vi "DetectCamera.vi"(8 "error in (no error)":errorcluster, 11 "Config In":T1) -> (0 "error out":errorcluster, 3 "Config Out":T1)   [LabVIEW 2019]
uses:
  Settings/Settings.ctl
  Support/Hardware Configuration.ctl
  Acquisition/Signal Type.ctl
  Logging/Logging Configuration.ctl
  Support/Camera Configuration.ctl
  E:/DevHardSoftware/MMicroscopy/HardwareAdapter/Camera/Dependencies/PVCamNET.dll
  Dependencies/PVCamNET.dll
  Acquisition/Acquisition.lvlib
  Logging/Logging.lvlib
  Settings/Settings.lvlib
panel:
  in  "Exposure time":dbl=30.0
  in  "stop":bool
  in  "start":bool
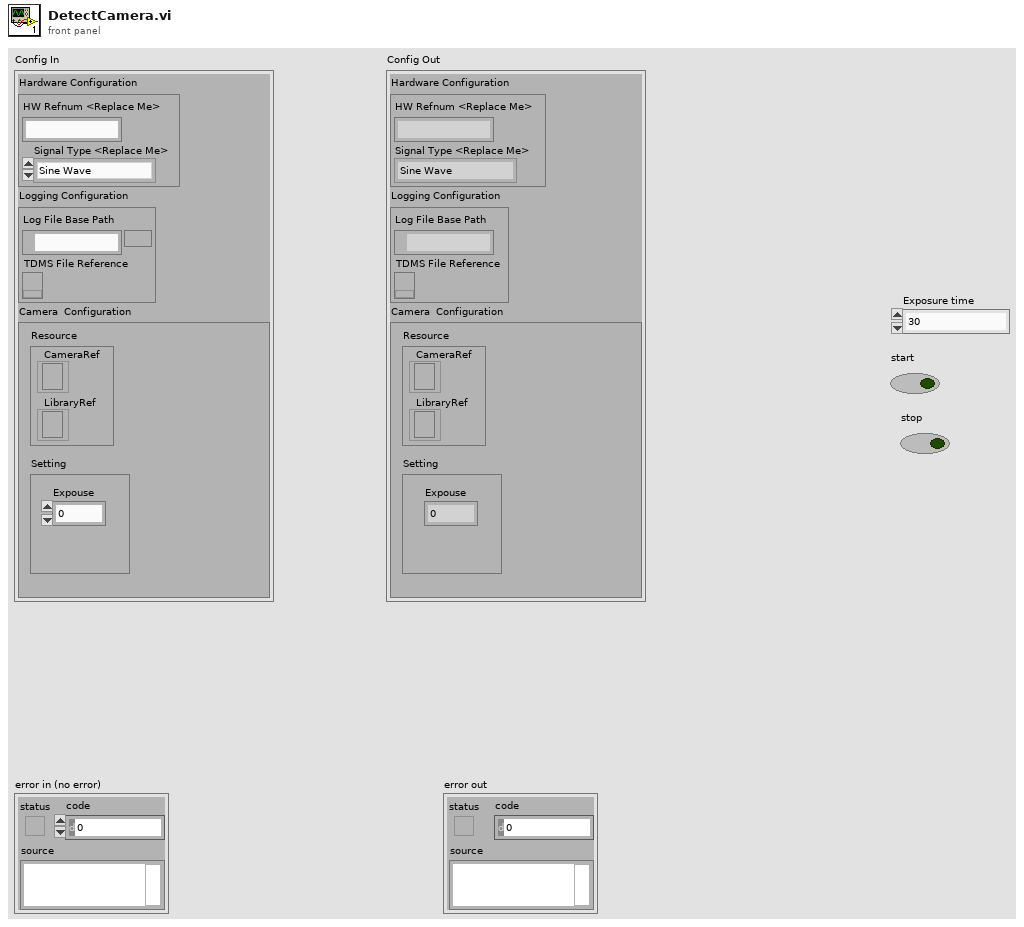
[diagram p1: front panel]
types:
  T1 = typedef "Settings.lvlib/Settings.ctl" = cluster{"Hardware Configuration":T2, "Logging Configuration":T4, "Camera Configuration":T5}
  T2 = typedef "Hardware Configuration.ctl" = cluster{"HW Refnum <Replace Me>":string, "Signal Type <Replace Me>":T3}
  T3 = typedef "Acquisition.lvlib/Signal Type.ctl" = enum16{"Sine Wave", "Square with Noise"}
  T4 = typedef "Logging.lvlib/Logging Configuration.ctl" = cluster{"Log File Base Path":path, "TDMS File Reference":refnum<k34>}
  T5 = typedef "Camera Configuration.ctl" = cluster{"Resource":cluster{"CameraRef":refnum<k24>, "LibraryRef":refnum<k24>}, "Setting":cluster{"Expouse":dbl}}
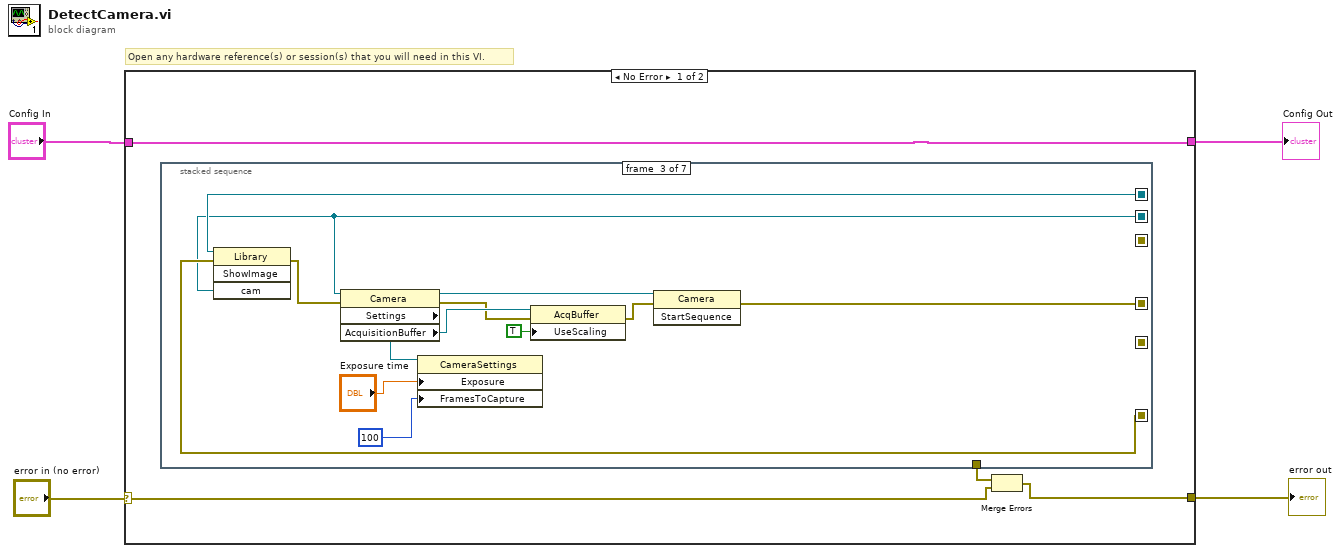
[diagram p0: block diagram]
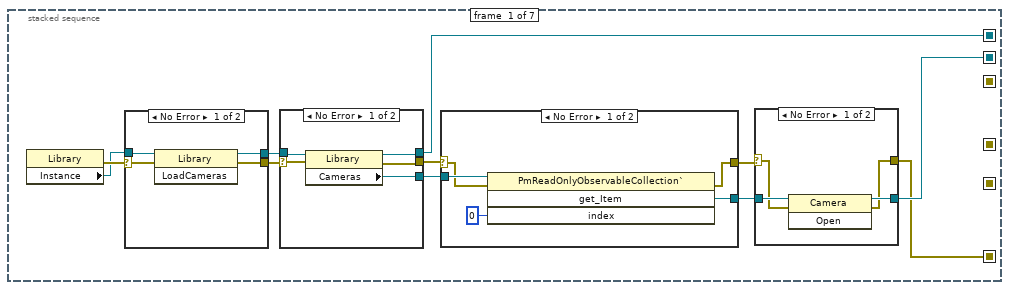
[diagram p2: hidden frame]
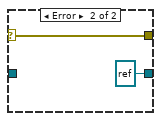
[diagram p3: hidden frame]
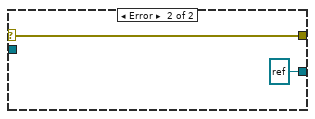
[diagram p4: hidden frame]
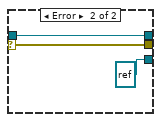
[diagram p5: hidden frame]
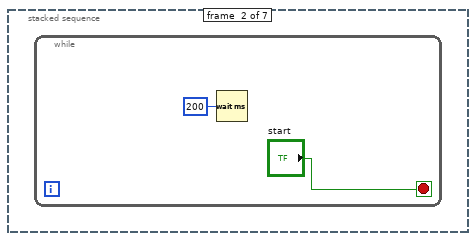
[diagram p7: hidden frame]
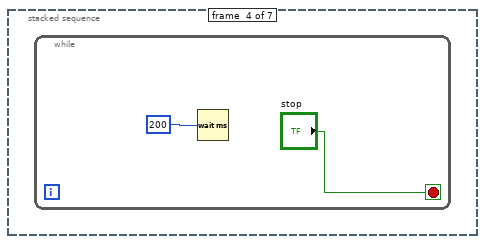
[diagram p8: hidden frame]
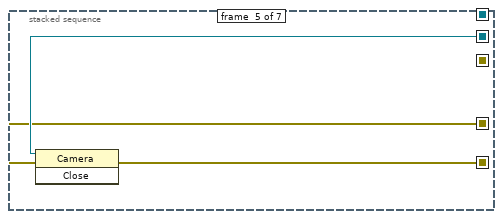
[diagram p9: hidden frame]
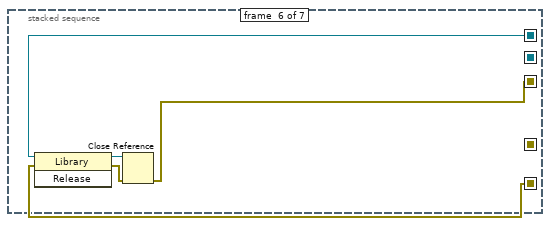
[diagram p10: hidden frame]
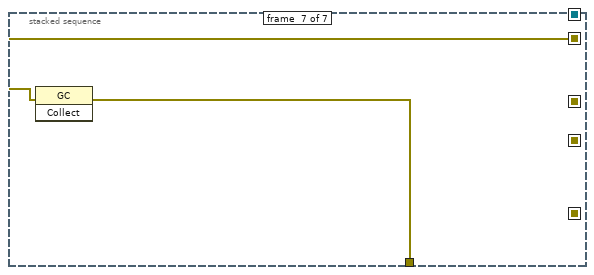
[diagram p11: hidden frame]
diagram:
  # "Open any hardware reference(s) or session(s) that you will need in this VI."
  n1 = case shown="No Error" "error in (no error)" {
    selector: "error in (no error)" -> [w6 w74]
    tunnel: [w5 w74] -> w3
    tunnel: "Config In" -> [w8 w75]
    tunnel: [w8 w75] -> w1
    frame No Error {
      n2 = stacked-sequence {
        seq-local: [w9 _ _ _ _ _ _] -> [_ _ w55 _ _ _ _]
        seq-local: [w10 _ _ _ _ _ _] -> [_ _ w53 _ w66 _ _]
        seq-local: [w11 _ _ _ _ _ _] -> [_ _ w61 _ _ w70 _]
        seq-local: [_ _ w49 _ _ _ _] -> [_ _ _ _ w65 _ _]
        seq-local: [_ _ _ _ w64 _ _] -> [_ _ _ _ _ w69 _]
        seq-local: [_ _ _ _ _ w67 _] -> [_ _ _ _ _ _ w73]
        tunnel: [_ _ _ _ _ _ w72] -> w7
        frame #0 {
          n3 = property class="Library"() -> (error out=w19:errorcluster, "Instance"=w16:refnum<k24>)  [unwired: 2 in, 1 out]
          n4 = case shown="No Error" w19 {
            selector: w19 -> [w42 w46]
            tunnel: [w43 w46] -> w17
            tunnel: [w44 w45] -> w18
            tunnel: w16 -> [w41 w45]
            frame No Error {
              n5 = invoke class="Library" method="LoadCameras"(reference=w41, error in=w42) -> (reference out=w44:refnum<k24>, error out=w43:errorcluster)  [unwired: 1 in, 1 out]
            }
            frame Error {
            }
          }
          n6 = case shown="No Error" w17 {
            selector: w17 -> [w37 w40]
            tunnel: [w34 w40] -> w13
            tunnel: w18 -> [w36 w39]
            tunnel: [w35 w39] -> w11
            tunnel: [w33 refnum<k24> refnum ("Cameras")] -> w15
            frame No Error {
              n7 = property class="Library"(reference=w36, error in=w37) -> (reference out=w35:refnum<k24>, error out=w34:errorcluster, "Cameras"=w33:refnum<k24>)
            }
            frame Error {
            }
          }
          n8 = case shown="No Error" w13 {
            selector: w13 -> [w27 w32]
            tunnel: w15 -> [w30 _]
            tunnel: [w28 refnum<k24> refnum ("get_Item")] -> w14
            tunnel: [w26 w32] -> w12
            frame No Error {
              n9 = invoke class="PmReadOnlyObservableCollection`" method="get_Item"(reference=w30, error in=w27, "index"=0) -> (error out=w26:errorcluster, "get_Item"=w28:refnum<k24>)  [unwired: 1 in, 2 out]
            }
            frame Error {
            }
          }
          n10 = case shown="No Error" w12 {
            selector: w12 -> [w21 w25]
            tunnel: [w20 w25] -> w9
            tunnel: w14 -> [w23 _]
            tunnel: [w22 refnum<k24> refnum ("get_Item")] -> w10
            frame No Error {
              n11 = invoke class="Camera" method="Open"(reference=w23, error in=w21) -> (reference out=w22:refnum<k24>, error out=w20:errorcluster)  [unwired: 1 in, 1 out]
            }
            frame Error {
            }
          }
        }
        frame #1 {
          n12 = while {
            stop <- "start" stop-if-true
            n13 = Wait (ms)(milliseconds to wait=u32 200) -> ()  [unwired: 1 out]
          }
        }
        frame #2 {
          n14 = invoke class="Library" method="ShowImage"(reference=w61, error in=w55, "cam"=w53) -> (error out=w54:errorcluster)  [unwired: 1 in, 3 out]
          n15 = property class="Camera"(reference=w53, error in=w54) -> (reference out=w52:refnum<k24>, error out=w51:errorcluster, "Settings"=w59:refnum<k24>, "AcquisitionBuffer"=w57:refnum<k24>)
          n16 = property class="CameraSettings"(reference=w59, "Exposure"="Exposure time", "FramesToCapture"=u16 100) -> ()  [unwired: 1 in, 2 out]
          n17 = property class="AcqBuffer"(reference=w57, error in=w51, "UseScaling"=TRUE) -> (error out=w50:errorcluster)  [unwired: 1 out]
          n18 = invoke class="Camera" method="StartSequence"(reference=w52, error in=w50) -> (error out=w49:errorcluster)  [unwired: 1 in, 2 out]
        }
        frame #3 {
          n19 = while {
            stop <- "stop" stop-if-true
            n20 = Wait (ms)(milliseconds to wait=u32 200) -> ()  [unwired: 1 out]
          }
        }
        frame #4 {
          n21 = invoke class="Camera" method="Close"(reference=w66, error in=w65) -> (error out=w64:errorcluster)  [unwired: 1 in, 2 out]
        }
        frame #5 {
          n22 = invoke class="Library" method="Release"(reference=w70, error in=w69) -> (reference out=w71:refnum<k24>, error out=w68:errorcluster)  [unwired: 1 in, 1 out]
          n23 = Close Reference(reference=w71, error in (no error)=w68) -> (error out=w67:errorcluster)
        }
        frame #6 {
          n24 = invoke class="GC" method="Collect"(error in=w73) -> (error out=w72:errorcluster)  [unwired: 2 in, 2 out]
        }
      }
      n25 = Merge Errors(w7, w6) -> (w5:errorcluster)
    }
    frame Error {
    }
  }
  "error out" <- w3
  "Config Out" <- w1
